vi "_IP Reporter.vi"(4 "ignore Gateway IP?(T)":bool=TRUE, 6 "Load From File(F)":bool, 8 "error in":errorcluster, 9 "WatchDog(notifier)":refnum<notifier>, 10 "Information":string, 11 "Setttings":T1={"address"="234.5.6.7", "receiver port"=58432, "Ignore Gateway IP"=TRUE, "HostName"=""}) -> (0 "error out":errorcluster)   [LabVIEW 2017]
doc: "Creates a write-only UDP multicast session and sends data to the specified port."
uses:
  _Typedef/Def-IniSettings -- Cluster.ctl
  _Typedef/Def-Report -- Cluster.ctl
  d1e7c7ed-84d8-4585-9177-9cc17e079b9e.vi
  <vilib>/Utility/error.llb/Clear Errors.vi
  <vilib>/Utility/libraryn.llb/Recursive File List.vi
  <userlib>/_OpenG.lib/lvdata/lvdata.llb/Set Data Name__ogtk.vi
  <vilib>/Utility/config.llb/Open Config Data.vi
  <userlib>/_OpenG.lib/variantconfig/variantconfig.llb/Write INI Cluster__ogtk.vi
  <userlib>/_OpenG.lib/variantconfig/variantconfig.llb/Read INI Cluster__ogtk.vi
  <vilib>/Utility/config.llb/Close Config Data.vi
  <vilib>/Utility/tcp.llb/UDP Multicast Write-Only Open.vi
panel:
  out "JSON string":string
  in  "Stop":bool
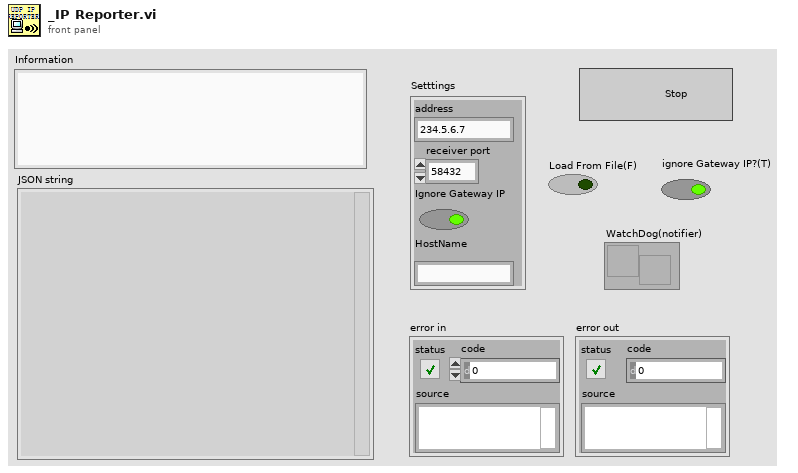
[diagram p1: front panel]
types:
  T1 = typedef "Def-IniSettings -- Cluster.ctl" = cluster{"address":string, "receiver port":u16, "Ignore Gateway IP":bool, "HostName":string}
  T2 = typedef "Def-Report -- Cluster.ctl" = cluster{"Host Name":string, "IPs":string[], "Timestamp":string, "Information":string}
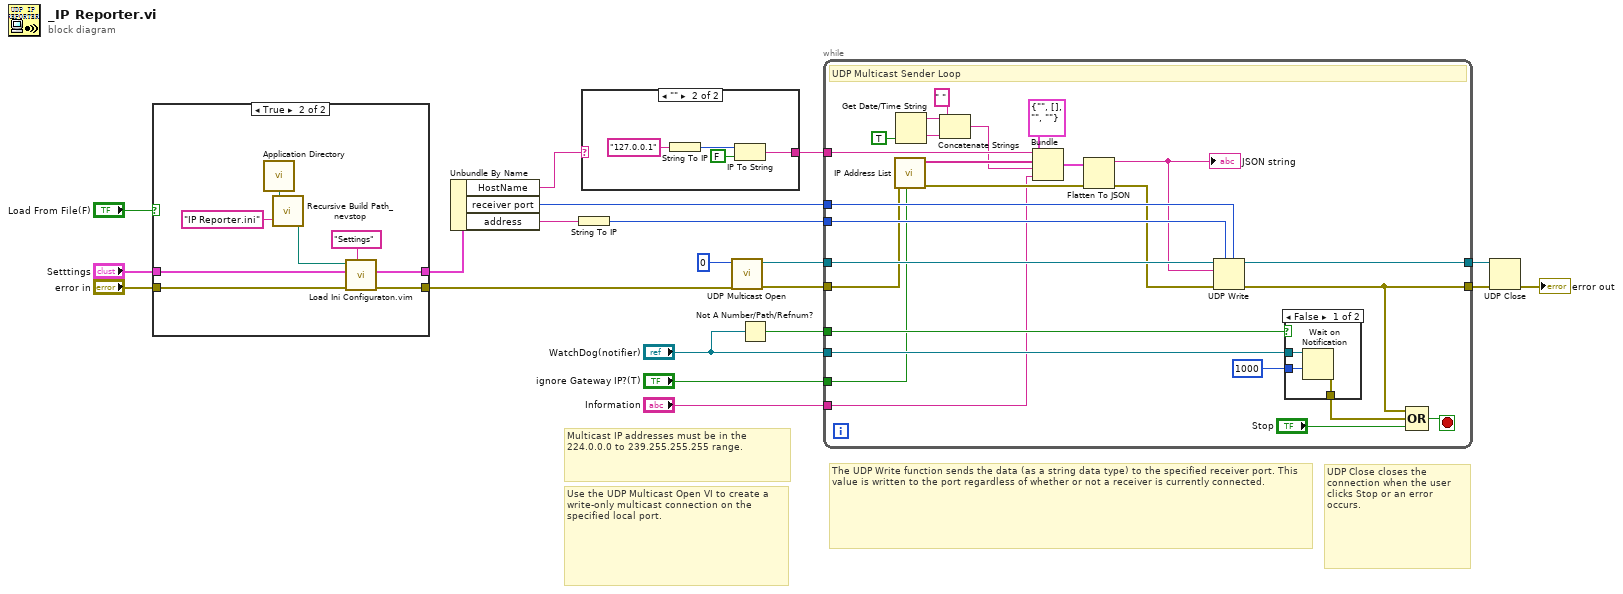
[diagram p0: block diagram]
diagram:
  # "UDP Close closes the connection when the user clicks Stop or an error occurs."
  # "Multicast IP addresses must be in the 224.0.0.0 to 239.255.255.255 range."
  # "The UDP Write function sends the data (as a string data type) to the specified receiver port. This value is written to the port regardless of whether or not a receiver is currently connected."
  # "Use the UDP Multicast Open VI to create a write-only multicast connection on the specified local port."
  n1 = case shown="True" "Load From File(F)" {
    tunnel: [w22 w30] -> w15
    tunnel: [w21 w29] -> w13
    tunnel: "Setttings" -> [w22 w25]
    tunnel: "error in" -> [w21 w24]
    frame False {
    }
    frame True {
      n2 = call <vilib>:"Application Directory.vi"() -> ("Application Directory"=w28:path)
      n3 = call <userlib>:"Recursive Build Path_nevstop.vi"("file name"="IP Reporter.ini", "Path"=w28) -> ("file path name"=w26:path)  [unwired: 1 in]
      n4 = call "Load Ini Configuraton.vim"("Session"="Settings", "error in (no error)"=w24, "Default Settings"=w25, "file path name"=w26) -> ("error out"=w29:errorcluster, "Settings out"=w30:T1)  [unwired: 6 in]
    }
  }
  n5 = Unbundle By Name(w15) -> ("HostName"=w10:string, "receiver port"=w12:u16, "address"=w14:string)
  n6 = String To IP(1:w14) -> (0:w18:u32)
  n7 = case shown="\"\"" w10 {
    selector: w10 -> [w31 _]
    tunnel: [w31 w35] -> w11
    frame "False", Default {
    }
    frame "" {
      n8 = String To IP(1:"127.0.0.1" ("name")) -> (0:w34:u32)
      n9 = IP To String(1:FALSE ("dot notation? (F)"), 2:w34) -> (0:w35:string)
    }
  }
  n10 = call-poly <vilib>:"UDP Multicast Open.vi"("error in (no error)"=w13, "port"=u16 0) -> ("error out"=w16:errorcluster, "connection ID"=w17:refnum<k16>)  [unwired: 8 in]
  n11 = Not A Number/Path/Refnum?(number/path/refnum="WatchDog(notifier)") -> (NaN/Path/Refnum?=w8:bool)
  n12 = while {
    tunnel: [w43] -> w19
    tunnel: w17 -> [w61]
    tunnel: w16 -> [w55]
    tunnel: [w58] -> w20
    tunnel: w18 -> [w57]
    tunnel: w12 -> [w56]
    tunnel: w11 -> [w48]
    tunnel: "WatchDog(notifier)" -> [w47]
    tunnel: w8 -> [w44]
    tunnel: "ignore Gateway IP?(T)" -> [w37]
    tunnel: "Information" -> [w36]
    stop <- w60 stop-if-true
    # "UDP Multicast Sender Loop"
    n13 = call "IP Address List.vi"("ignore Gateway IP?"=w37, "error in (no error)"=w55) -> ("error out"=w54:errorcluster, "Array"=w50:string[])  [unwired: 8 in]
    n14 = Get Date/Time String(want seconds? (F)=TRUE) -> (date string=w42:string, time string=w41:string)  [unwired: 2 in]
    n15 = Concatenate Strings(w42, " " ("string"), w41) -> (w39:string)
    n16 = Bundle(cluster=T2 {"Host Name"="", "IPs"=[], "Timestamp"="", "Information"=""} ("Pack"), "Host Name"=w48, "IPs"=w50, "Timestamp"=w39, "Information"=w36) -> (w49:T2)
    n17 = Flatten To JSON(anything=w49, error in (no error)=w54) -> (JSON string=w52:string, 11:w53:errorcluster)  [unwired: 1 in]
    "JSON string" <- w52
    n18 = UDP Write(address=w57, port or service name=w56, connection ID=w61, data in=w52, 8:w53) -> (error out=w43:errorcluster, 3:w58:refnum<k16>)  [unwired: 1 in]
    n19 = case shown="False" w44 {
      tunnel: w47 -> [w64 _]
      tunnel: 1000 ("timeout in ms (-1)") -> [w63 _]
      tunnel: [w62 _] -> w45
      frame False {
        n20 = Wait on Notification(notifier=w64, timeout in ms (-1)=w63) -> (error out=w62:errorcluster)  [unwired: 2 in, 3 out]
      }
      frame True {
      }
    }
    n21 = Compound Arithmetic op=OR(w43, w45, "Stop") -> (w60:bool)
  }
  n22 = UDP Close(connection ID=w20, 8:w19) -> (error out=→"error out":errorcluster)  [unwired: 1 out]
